vi "Data JSON.vi"(8 "error in (no error)":errorcluster, 11 "Request in":refnum<class "Request.lvclass">) -> (0 "error out":errorcluster, 2 "Data JSON":string, 3 "Request out":refnum<class "Request.lvclass">)   [LabVIEW 2022 SP3, in "obs-websocket-lv.lvlib" / "Request.lvclass"]
uses:
  Request.lvclass
  Request.lvclass/Request.ctl
  <vilib>/IlluminatedG/lv-web-crypto/lv-json/JSON/JSON.lvlib
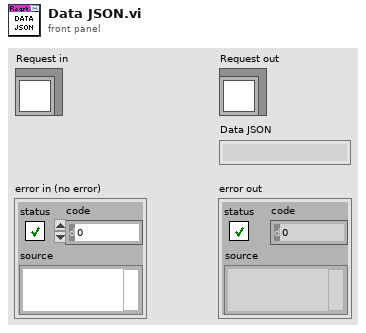
[diagram p1: front panel]
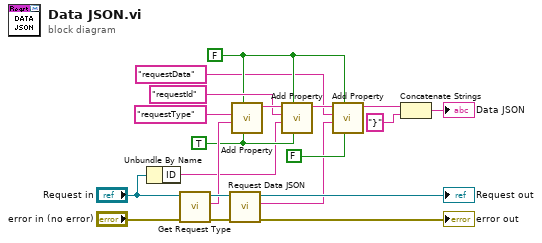
[diagram p0: block diagram]
diagram:
  w7 = FALSE ("Include Empty?")
  w11 = TRUE ("String?")
  n1 = Unbundle By Name("Request in") -> ("ID"=w9:string)
  n2 = call-dynamic "Get Request Type.vi"("error in (no error)"="error in (no error)", "Request in"="Request in") -> ("error out"=w18:errorcluster, "Request Type"=w13:string, "Request out"=w19:refnum<class "Request.lvclass">)  [unwired: 7 in]
  n3 = call-dynamic "Request Data JSON.vi"("error in (no error)"=w18, "Request in"=w19) -> ("error out"=→"error out":errorcluster, "Request Data JSON"=w4:string, "Request out"=→"Request out":refnum<class "Request.lvclass">)  [unwired: 7 in]
  n4 = call <vilib>:"Add Property.vi"("String?"=w11, "Include Empty?"=w7, "Value"=w13, "Property Name"="requestType") -> ("String out"=w12:string)  [unwired: 7 in]
  n5 = call <vilib>:"Add Property.vi"("String?"=w11, "Include Empty?"=w7, "Value"=w9, "Property Name"="requestId", "String In"=w12) -> ("String out"=w8:string)  [unwired: 6 in]
  n6 = call <vilib>:"Add Property.vi"("String?"=FALSE, "Include Empty?"=w7, "Value"=w4, "Property Name"="requestData", "String In"=w8) -> ("String out"=w3:string)  [unwired: 6 in]
  n7 = Concatenate Strings(w3, "}" ("string")) -> (→"Data JSON":string)
